vi "Pre Launch Init.vi"(11 "Acquisition UI in":refnum<class "Acquisition UI.lvclass">) -> (0 "error out":errorcluster, 3 "Acquisition UI out":refnum<class "Acquisition UI.lvclass">)   [LabVIEW 2018, in "Acquisition UI.lvlib" / "Acquisition UI.lvclass"]
doc: "(<B>Filename</B>: Actor Framework.lvlib:Actor.lvclass:Pre Launch Init.vi)\n\nDefines behavior that occurs after the Launch Nested Actor method is invoked but before the actor's Actor Core method begins running.\n\nBy default, this method does nothing. A descendant class may override it to define behavior."
uses:
  Acquisition UI.lvclass
  <vilib>/ActorFramework/Actor/Actor.lvclass
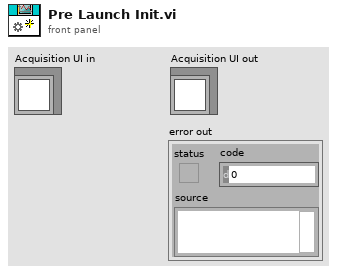
[diagram p1: front panel]
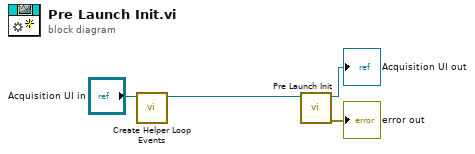
[diagram p0: block diagram]
diagram:
  n1 = call "Create Helper Loop Events.vi"("Acquisition UI in"="Acquisition UI in") -> ("Acquisition UI out"=w1:refnum<class "Acquisition UI.lvclass">)  [unwired: 10 in]
  n2 = call-parent "Pre Launch Init.vi"("Actor in"=w1) -> ("error out"=→"error out":errorcluster, "Actor out"=→"Acquisition UI out":refnum<class "Acquisition UI.lvclass">)  [unwired: 9 in]
